vi "xiC - IMAQ - PRMErrorHandler.vi"(6 "PRM.Desc.":string, 8 "error in (no error)":errorcluster, 11 "Attributes In":T1) -> (0 "error out":errorcluster, 3 "Attributes Out":T1)   [LabVIEW 2013]
uses:
  xiC - IMAQ - Attributes.ctl
  C:/Projects/Cameras3.x/xiLib/xiLIB_64bit/xiLIB/xiCamLib/API/x64/xiApi.NETX64.dll
  xiLIB_64bit/xiLIB/xiCamLib/API/x64/xiApi.NETX64.dll
  xiC - IMAQ - TreeDisplayType.ctl
  xiC - IMAQ - Globals.vi
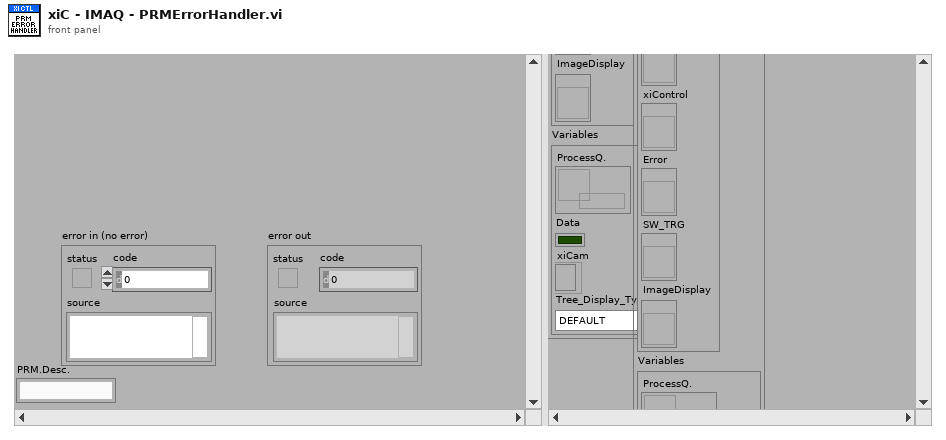
[diagram p1: front panel]
types:
  T1 = typedef "xiC - IMAQ - Attributes.ctl" = cluster{"Controls":cluster{"VI Ref.":refnum<vi>, "Tree":refnum<vi>, "Info":refnum<vi>, "PRMName":refnum<vi>, "xiControl":refnum<vi>, "Error":refnum<vi>, "SW_TRG":refnum<vi>, "ImageDisplay":refnum<vi>}, "Variables":cluster{"ProcessQ.":refnum<queue>, "Data":bool, "xiCam":refnum<k24>, "Tree_Display_Type":T2}}
  T2 = typedef "xiC - IMAQ - TreeDisplayType.ctl" = enum16{"DEFAULT", "HIDE_MAX_MIN"}
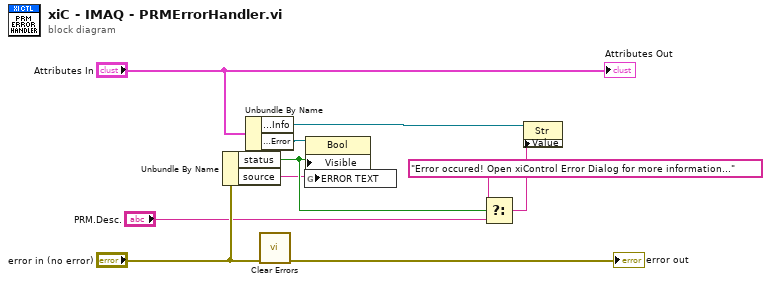
[diagram p0: block diagram]
diagram:
  n1 = Unbundle By Name("error in (no error)") -> ("status"=w5:bool, "source"=w3:string)
  n2 = Unbundle By Name("Attributes In") -> ("Controls.Info"=w9:refnum<vi>, "Controls.Error"=w10:refnum<vi>)
  n3 = call <vilib>:"Clear Errors.vi"("error in (no error)"="error in (no error)") -> ("error out"=→"error out":errorcluster)  [unwired: 6 in]
  n4 = global write "xiC - IMAQ - Globals.vi" "ERROR TEXT"(w3) -> ()
  n5 = property class="Bool"(reference=w10, "Visible"=w5) -> ()  [unwired: 1 in, 2 out]
  n6 = Select(t="Error occured! Open xiControl Error Dialog for more information...", s=w5, f="PRM.Desc.") -> (s? t:f=w4:string)
  n7 = property class="Str"(reference=w9, "Value"=w4) -> ()  [unwired: 1 in, 2 out]
  "Attributes Out" <- "Attributes In"
